vi "rszvl_core_global.vi"() -> ()   [LabVIEW 2014]
panel:
  in  "Supported Models":string[](array[string])=["ZVL", "ZNL"]
  in  "Repeated Capabilities":T1(array[cluster])=[{"repCapName"="Marker", "identifiers"=["M1", "M2", "M3", "M4"], "cmdValues"=["1", "2", "3", "4"]}, {"repCapName"="Default", "identifiers"=["DEF1", "DEF2", "DEF3"], "cmdValues"=["1", "2", "3"]}, {"repCapName"="Destination", "identifiers"=["DE1", "DE2"], "cmdValues"=["1", "2"]}, {"repCapName"="CMAP", "identifiers"=["CM1", "CM2", "CM3", "CM4", "CM5", "CM6", "CM7", "CM8", "CM9", "CM10", "CM11", "CM12", "CM13", "CM14", "CM15", "CM16", "CM17", "CM18", "CM19", "CM20", "CM21", "CM22", "CM23", "CM24", "CM25", "CM26", "CM27"], "cmdValues"=["1", "2", "3", "4", "5", "6", "7", "8", "9", "10", "11", "12", "13", "14", "15", "16", "17", "18", "19", "20", "21", "22", "23", "24", "25", "26", "27"]}, {"repCapName"="Limit", "identifiers"=["L1", "L2", "L3", "L4", "L5", "L6", "L7", "L8"], "cmdValues"=["1", "2", "3", "4", "5", "6", "7", "8"]}, {"repCapName"="DeltaMarker", "identifiers"=["DM1", "DM2", "DM3", "DM4"], "cmdValues"=["1", "2", "3", "4"]}, {"repCapName"="Trace", "identifiers"=["TR1", "TR2", "TR3", "TR4", "TR5", "TR6", "TR7", "TR8", "TR9", "TR10", "TR11", "TR12", "TR13", "TR14", "TR15", "TR16", "TR17", "TR18", "TR19", "TR20"], "cmdValues"=["1", "2", "3", "4", "5", "6", "7", "8", "9", "10", "11", "12", "13", "14", "15", "16", "17", "18", "19", "20"]}, {"repCapName"="Line", "identifiers"=["L1", "L2"], "cmdValues"=["1", "2"]}, {"repCapName"="Channel", "identifiers"=["CH1", "CH2", "CH3", "CH4", "CH5", "CH6", "CH7", "CH8", "CH9", "CH10", "CH11", "CH12", "CH13", "CH14", "CH15", "CH16", "CH17", "CH18", "CH19", "CH20"], "cmdValues"=["1", "2", "3", "4", "5", "6", "7", "8", "9", "10", "11", "12", "13", "14", "15", "16", "17", "18", "19", "20"]}, {"repCapName"="StatisticMeasType", "identifiers"=["StatMean", "StatPeak", "StatCrestFactor"], "cmdValues"=["MEAN", "PEAK", "CFAC"]}, {"repCapName"="DiagramArea", "identifiers"=["DA1", "DA2", "DA3", "DA4", "DA5", "DA6", "DA7", "DA8", "DA9", "DA10"], "cmdValues"=["1", "2", "3", "4", "5", "6", "7", "8", "9", "10"]}, {"repCapName"="Segment", "identifiers"=["SEG1", "SEG2", "SEG3", "SEG4", "SEG5", "SEG6", "SEG7", "SEG8", "SEG9", "SEG10", "SEG11", "SEG12", "SEG13", "SEG14", "SEG15", "SEG16", "SEG17", "SEG18", "SEG19", "SEG20"], "cmdValues"=["1", "2", "3", "4", "5", "6", "7", "8", "9", "10", "11", "12", "13", "14", "15", "16", "17", "18", "19", "20"]}, {"repCapName"="Port", "identifiers"=["P1", "P2", "P3", "P4", "P5", "P6", "P7", "P8", "P9", "P10"], "cmdValues"=["1", "2", "3", "4", "5", "6", "7", "8", "9", "10"]}, {"repCapName"="NWAMarker", "identifiers"=["MAR1", "MAR2", "MAR3", "MAR4", "MAR5", "MAR6", "MAR7", "MAR8", "MAR9", "MAR10"], "cmdValues"=["1", "2", "3", "4", "5", "6", "7", "8", "9", "10"]}, {"repCapName"="FMOffsetResult", "identifiers"=["FMOffImm", "FMOffAver"], "cmdValues"=["IMM", "AVER"]}, {"repCapName"="ResultDetector", "identifiers"=["ResDetPosPeak", "ResDetNegPeak", "ResDetAverPeak", "ResDetRMS"], "cmdValues"=["PPE", "MPE", "MIDD", "RMS"]}, {"repCapName"="ModifStopStart", "identifiers"=["Stop", "Start"], "cmdValues"=["STOP", "START"]}, {"repCapName"="WiMSegment", "identifiers"=["WSEG1", "WSEG2", "WSEG3"], "cmdValues"=["1", "2", "3"]}, {"repCapName"="Bitmap", "identifiers"=["B1", "B2", "B3", "B4", "B5", "B6", "B7", "B8", "B9", "B10", "B11", "B12", "B13", "B14", "B15", "B16", "B17", "B18"], "cmdValues"=["1", "2", "3", "4", "5", "6", "7", "8", "9", "10", "11", "12", "13", "14", "15", "16", "17", "18"]}, {"repCapName"="Zone", "identifiers"=["Z1", "Z2", "Z3", "Z4", "Z5", "Z6", "Z7", "Z8", "Z9", "Z10", "Z11", "Z12", "Z13", "Z14", "Z15", "Z16", "Z17", "Z18", "Z19", "Z20", "Z21", "Z22", "Z23", "Z24", "Z25", "Z26"], "cmdValues"=["1", "2", "3", "4", "5", "6", "7", "8", "9", "10", "11", "12", "13", "14", "15", "16", "17", "18", "19", "20", "21", "22", "23", "24", "25", "26"]}, {"repCapName"="Burst", "identifiers"=["BU1", "BU2", "BU3", "BU4", "BU5", "BU6", "BU7", "BU8", "BU9", "BU10", "BU11", "BU12", "BU13", "BU14", "BU15", "BU16", "BU17", "BU18", "BU19", "BU20", "BU21", "BU22", "BU23", "BU24", "BU25", "BU26", "BU27", "BU28", "BU29", "BU30", "BU31", "BU32"], "cmdValues"=["1", "2", "3", "4", "5", "6", "7", "8", "9", "10", "11", "12", "13", "14", "15", "16", "17", "18", "19", "20", "21", "22", "23", "24", "25", "26", "27", "28", "29", "30", "31", "32"]}, {"repCapName"="AnalogModulation", "identifiers"=["AnalogAM", "AnalogFM", "AnalogPM"], "cmdValues"=["AM", "FM", "PM"]}, {"repCapName"="BtoRtpTimePacketSection", "identifiers"=["SECTION_TIME_GFSK", "SECTION_TIME_DPSK"], "cmdValues"=["GAV", "DAV"]}, {"repCapName"="ModifMinMaxAver", "identifiers"=["Min", "Max", "Aver"], "cmdValues"=["MIN", "MAX", "AVER"]}, {"repCapName"="Frequency", "identifiers"=["F1", "F2"], "cmdValues"=["1", "2"]}, {"repCapName"="ModifLowUpp", "identifiers"=["Low", "Upp"], "cmdValues"=["LOW", "UPP"]}, {"repCapName"="BtoRtpPacketSection", "identifiers"=["SECTION_GFSK", "SECTION_DPSK"], "cmdValues"=["GFSK", "DPSK"]}, {"repCapName"="ModifAboveBelow", "identifiers"=["Peak", "Above", "Below", "Next"], "cmdValues"=["PEAK", "ABOV", "BEL", "NEXT"]}, {"repCapName"="InputOutput", "identifiers"=["Inp", "Out"], "cmdValues"=["INP", "OUTP"]}, {"repCapName"="NoiseTraceMemory", "identifiers"=["MEM1", "MEM2", "MEM3"], "cmdValues"=["1", "2", "3"]}, {"repCapName"="Alternate", "identifiers"=["A1", "A2", "A3", "A4"], "cmdValues"=["1", "2", "3", "4"]}, {"repCapName"="3GPPChannel", "identifiers"=["Cpich", "Pccpch"], "cmdValues"=["CPIC", "PCCP"]}, {"repCapName"="WiMAXBurstMeasurement", "identifiers"=["Carrier", "Burst", "Symbol"], "cmdValues"=["CARR", "BURS", "SYMB"]}, {"repCapName"="WiMAXMeasurement", "identifiers"=["Constellation", "Bitstream"], "cmdValues"=["CONS", "STAT:BSTR"]}, {"repCapName"="Window", "identifiers"=["Win1", "Win2"], "cmdValues"=["1", "2"]}, {"repCapName"="AtvCarrier", "identifiers"=["CN", "CSO", "CTB"], "cmdValues"=["CN", "CSO", "CTB"]}, {"repCapName"="AtvSoundCarrier", "identifiers"=["SC1", "SC2"], "cmdValues"=["S1", "S2"]}, {"repCapName"="AtvVisionModulResult", "identifiers"=["VisCarrPow", "ResPicture", "Depth"], "cmdValues"=["VCP", "RPC", "MDEP"]}, {"repCapName"="AtvCarrierResult", "identifiers"=["RefPow", "NoiseFloorCorr", "FreqRel", "CR", "NoiseRefBw"], "cmdValues"=["RPOW", "NFC", "MFR", "", "NRBW"]}, {"repCapName"="DtvErrorMeas", "identifiers"=["EVMPeak", "EVMRms", "MERPeak", "MERRms"], "cmdValues"=["EVMP", "EVMR", "MERP", "MERR"]}, {"repCapName"="DtvShoulderAtt", "identifiers"=["SAttLow", "SAttUpp"], "cmdValues"=["SAL", "SAUP"]}]
  in  "Attributes":T2(array[cluster])=[{"Level"=1, "Descriptive Name"="Basic Operation", "Class Only"=TRUE, "Data Type"=0, "Access"=0, "Identifier"="", "Range Table"="", "Command"="", "Read Callback"="", "Write Callback"="", "Range Callback"="", "Check Callback"="", "Rngtable Callback"="", "Coerce Callback"="", "User Callback"="", "Supported Models"="", "Instrument Options"="", "Repeated Capabilities"="", "Restricted Repeated Capabilities"="", "Help"="(1) Amplitude Units:\nSpecifies the amplitude units for input, output and display amplitude.\n\n(2) Instrument Mode:\nThis attribute switches between the measurement modes by means of text parameters.\n\n(3) Attenuation:\nThis attribute sets the input attenuator. To protect the input mixer against damage from overloads, the setting 0 dB can be obtained by entering numerals, not by using the command DEC.\nThe attenuation can be set in 5 dB steps. If the defined reference level cannot be set for the set RF attenuation, the reference level will be adjusted accordingly.\nIn the default state with Spectrum Analyzer mode, the attenuation set on the step attenuator is coupled to the reference level of the instrument. If the attenuation is programmed directly, the coupling to the reference level is switched off.\n\n(4) Attenuation Auto:\nEnables or disables auto attenuation.\n\n(5) Frequency Start:\nSpecifies the left edge of the frequency domain in Hertz. This is used in conjunction with the RSZVL_ATTR_FREQUENCY_STOP Stop attribute to define the frequency domain. If the RSZVL_ATTR_FREQUENCY_START attribute value is equal to the RSZVL_ATTR_FREQUENCY_STOP attribute value then the spectrum analyzers horizontal attributes are in time-domain.\n\n(6) Frequency Stop:\nSpecifies the right edge of the frequency domain in Hertz. This is used in conjunction with the RSZVL_ATTR_FREQUENCY_START attribute to define the frequency domain. If the RSZVL_ATTR_FREQUENCY_START attribute value is equal to the RSZVL_ATTR_FREQUENCY_STOP attribute value then the spectrum analyzers horizontal attributes are in time-domain.\n\n(7) Frequency Offset:\nThis attribute sets the frequency offset of the instrument.\n\n(8) Center Frequency:\nThe attribute defines the center frequency of the analyzer or the measuring frequency for span = 0.\n\n(9) Center Frequency Step:\nThis attribute defines the step width of the center frequency.\n\n(10) Center Frequency Step Auto:\nThis attribute couples the step size of the center frequency to the span (ON) or sets the value of the center frequency entered via [SENSe<1|2>:]FREQuency:CENTer:STEP (OFF).\n\n(11) Center Frequency Coupling:\nThis attribute couples the step width of the center frequency to span (span >0) or to the resolution bandwidth (span = 0) or cancels the couplings.\n\n(12) Center Frequency Coupling Factor:\nThis attribute couples the step width of the center frequency with a factor to the span (span >0) or to the resolution bandwidth (span = 0).\n\n(13) Frequency Span:\nThis attribute defines the frequency span in the analyzer mode.\n\n(14) Full Frequency Span:\nThis attribute sets the frequency span in the analyzer mode to its maximum.\n\n(15) Frequency Mode:\nThis attribute switches between frequency domain (SWEep) and time domain (CW | FIXed) in the analyzer mode. For CW and FIXed, the frequency setting is via command FREQuency:CENTer. In the SWEep mode, the setting is via commands FREQuency:STARt, STOP, CENTer and SPAN.\n\n(16) Input Impedance:\nThis attribute the nominal input impedance of the instrument. The set impedance is taken into account in all level indications of results.\n\n(17) Number of Sweeps:\nThis attribute defines the number of sweeps started with single sweep, which are used for calculating the average or maximum value. In average mode, the value 0 defines a continuous averaging of measurement data over 10 sweeps.\n\n(18) Reference Level:\nThis attribute configures the reference level for the signal analyzer mode.\n\n\n(19) Reference Level Offset:\nThis attribute defines the offset of the reference level.\n\n(20) Resolution Bandwidth:\nThis attribute defines the analyzer's resolution bandwidth.\n\n(21) Resolution Bandwidth Auto:\nIn SPECTRUM mode, this attribute either automatically couples the resolution bandwidth of the instrument to the span or cancels the coupling.\nIn FM DEMOD mode, this attribute either automatically couples the IF bandwidth of the instrument to the demodulation bandwidth or cancels the coupling (BWRBW = 10 * BWDemod).\nIn FM DEMOD mode, the coupling refers to the demodulation bandwidth (BWRBW = 10 * BWDemod). The automatic coupling adapts the resolution bandwidth to the currently set frequency span according to the relationship between frequency span and resolution bandwidth. The 6 dB bandwidths 200 Hz, 9 kHz and 120 kHz and the channel filters available from Version 1.10 are not set by the automatic coupling.\n\nNote: This attribute is not available for GSM/EDGE measurements modulation accuracy (MAC), phase/frequency error (PFE) and power versus time (PVT). During these measurements the bandwidth is selected due to GSM standard.\n\n(22) Resolution Bandwidth Ratio:\nThis attribute defines the ratio resolution bandwidth (Hz) / span (Hz). The ratio to be entered is reciprocal to the ratio span/RBW used in manual control.\n\n(23) Sweep Mode:\nThis attribute determines whether the trigger system is continuously initiated (continuous) or performs single measurements (single).\nIn the spectrum analysis mode, this setting refers to the sweep sequence (switching between continuous/single sweep).\n\n(24) Sweep Time:\nThis attribute defines the sweep time.\n\n(25) Sweep Time Auto:\nThis attribute controls the automatic coupling of the sweep time to the frequency span and bandwidth settings.\n\n(26) Sweep Points:\nThis attribute defines the number of measurement points for one sweep run.\n\n(27) Get Sweep Count Current:\nThis attribute returns the current number of started sweeps. A sweep count value should be set and the device should be in single sweep mode.\n\n(28) Vertical Scale:\nThis attribute toggles between linear and logarithmic display.\n\n(29) Video Bandwidth:\nThis attribute defines the instrument's video bandwidth.\n\n(30) Video Bandwidth Auto:\nThis attribute either automatically couples the instrument's video bandwidth to the resolution bandwidth or cancels the coupling.\n\n(31) Video Bandwidth Ratio:\nThis attribute defines the ratio video bandwidth (Hz) / resolution bandwidth (Hz). The ratio to be entered is reciprocal to the ratio RBW/VBW used in manual control.\n\n(32) Low-Level Measurement (Class):\nThis class contains attributes for initiate and abort measurement.\n\n(1) Abort:\nThis attribute aborts a current measurement and resets the trigger system.\n\n(2) Initiate:\nThis attribute initiates a new sweep.\nIn single sweep mode, synchronization to the end of the indicated number of measurements is achieved with the command *OPC. In continuous-sweep mode, synchronization to the sweep end is not possible since the overall measurement never ends.\n\n(3) Initiate Continuous:\nThis attribute determines whether the trigger system is continuously initiated (continuous) or performs single measurements (single).\nIn the spectrum analysis mode, this setting refers to the sweep sequence (switching between continuous/single sweep).\n\n(4) Send Software Trigger:\nThis attribute sends a software trigger to the instrument.\n\n(5) Continue Measurement:\nThis attribute continues a stopped measurement at the current position in single sweep mode. The function is useful especially for trace functions MAXHold, MINHold and AVERage if the previous results are not to be cleared with Sweep Count > 0 or Average Count > 0 on restarting the measurement (INIT:IMMediate resets the previous results on restarting the measurement).\nThe single-sweep mode is automatically switched on. Synchronization to the end of the indicated number of measurements can then be performed with the command *OPC, *OPC? or *WAI. In the continuous-sweep mode, synchronization to the sweep end is not possible since the overall measurement never ends.\n\n\n\n(33) Average (Class):\nThis subsystem calculates the average of the acquired data.\n\n(1) Averaging State:\nThis attribute switches on or off the average calculation for the selected trace.\n\n(2) Averaging Type:\nThis attribute selects the type of average function. If Video is selected, the logarithmic power is averaged and, if Linear is selected, the power values are averaged before they are converted to logarithmic values. The type of average calculation is equally set for all traces\n\n(3) Averaging Count:\nThis attribute defines the number of measurements which contribute to the average value.\nIt should be noted that continuous averaging will be performed after the indicated number has been reached in continuous sweep mode.\nIn single sweep mode, the sweep is stopped as soon as the indicated number of measurements (sweeps) is reached. Synchronization to the end of the indicated number of measurements is only possible in single sweep mode.\n\n(4) Averaging Count Auto:\nThis attribute is implemented only for reasons of compatibility with the FSP family. It selects a suitable number of counts for the selected measurement type.\n\n\n\n(34) Bandwidth (Class):\nThis class contains attributes configuring resolution and video bandwidth.\n\n(1) Resolution Bandwidth Filter Type:\nThis attribute sets the filter type for the resolution bandwidth.\n\n(2) Video Bandwidth Filter Type:\nThis attribute selects the position of the video filter in the signal path, provided that the resolution bandwidth is <=100 kHz:\n\n(35) Trace (Class):\nTrace settings and configuration.\n\n(1) Trace State:\nThis attribute switches on or off the display of the corresponding trace.\n\n(2) Trace Reset Behavior:\nThis attribute specifies whether or not the traces with peak or minimum value detection are reset after specific parameter changes.\n\n(3) Trace Type:\nThis attribute defines the type of display and the evaluation of the traces. WRITE corresponds to the Clr/Write mode of manual operation. The trace is switched off (= BLANK in manual operation) with DISP:WIND:TRAC:STAT OFF.\n\n(4) Trace Math State:\nThis attribute switches the mathematical relation of traces on or off.\n\n(5) Trace Math Position:\nThis attribute defines the position of the result of the trace mathematics. The indication is in % of the screen height, with 100% corresponding to the upper diagram border.\n\n(6) Detector Type:\nSpecifies the detection method used to capture and process the signal. This governs the data acquisition for a particular sweep, but does not have any control over how multiple sweeps are processed.\n\n(7) Detector Type Auto:\nEnables the auto detector.\n\n(36) Calibration (Class):\n(1) Calibration:\nThis attribute initiates the acquisition of system error correction data. A 0 is returned if the acquisition was successful.\n\n(2) Calibration Abort:\nThis atribute aborts the acquisition of correction data and restores the last complete correction data set.\n\n(3) Calibration Result Query:\nThis attribute outputs the results of the correction data acquisition.\n\n(4) Calibration State:\nThis attribute determines whether the current calibration data are taken into account by the instrument (ON) or not (OFF).\n\n\n\n(37) User Port (Class):\n(1) User Ports State:\nThis attribute toggles the control lines of the user ports between INPut and OUTPut. With ON, the user port is switched to INPut, with OFF to OUTPut.\n\n(2) User Ports Control Lines:\nThis attribute queries the control lines of the user ports.\n\n(3) User Ports Output Control Lines:\nThis attribute sets the control lines of the user ports. The user port is written to with the given binary pattern. If the user port is programmed to INPut instead of OUTPut, the output value is temporarily stored.", "Flags"={"OPC Wait"=FALSE, "Dont check status"=FALSE, "*WAI"=FALSE}, "Check Status Callback"=""}, {"Level"=2, "Descriptive Name"="Amplitude Units", "Class Only"=FALSE, "Data Type"=0, "Access"=2, "Identifier"="RSZVL_ATTR_AMPLITUDE_UNITS", "Range Table"="rszvl_rngAmplitudeUnitsRangeTable", "Command"="UNIT:POW", "Read Callback"="", "Write Callback"="", "Range Callback"="", "Check Callback"="", "Rngtable Callback"="", "Coerce Callback"="", "User Callback"="", "Supported Models"="", "Instrument Options"="", "Repeated Capabilities"="", "Restricted Repeated Capabilities"="", "Help"="Specifies the amplitude units for input, output and display amplitude.\n\nAvailable Repeated Capabilities:\nNone\n\nRemote-control command(s):\nUNIT<1|2>:POWer DBM | DBPW | WATT | DBUV | DBMV | VOLT | DBUA | AMPere", "Flags"={"OPC Wait"=FALSE, "Dont check status"=FALSE, "*WAI"=FALSE}, "Check Status Callback"=""}, {"Level"=2, "Descriptive Name"="Instrument Mode", "Class Only"=FALSE, "Data Type"=0, "Access"=2, "Identifier"="RSZVL_ATTR_INSTR_MODE", "Range Table"="rszvl_rngInstrMode", "Command"="INST:SEL", "Read Callback"="", "Write Callback"="", "Range Callback"="", "Check Callback"="", "Rngtable Callback"="", "Coerce Callback"="", "User Callback"="", "Supported Models"="", "Instrument Options"="", "Repeated Capabilities"="", "Restricted Repeated Capabilities"="", "Help"="This attribute switches between the measurement modes by means of text parameters.\n\nAvailable Repeated Capabilities:\nNone\n\nRemote-control command(s):\nINSTrument[:SELect] NWA | SAN | NOISe | BWCD | WLAN | WiMAX | ADEM | BTO | CATV", "Flags"={"OPC Wait"=FALSE, "Dont check status"=FALSE, "*WAI"=FALSE}, "Check Status Callback"=""}, {"Level"=2, "Descriptive Name"="Attenuation", "Class Only"=FALSE, "Data Type"=1, "Access"=2, "Identifier"="RSZVL_ATTR_ATTENUATION", "Range Table"="rszvl_rngAttenuationRangeTable", "Command"="INP:ATT", "Read Callback"="", "Write Callback"="", "Range Callback"="", "Check Callback"="", "Rngtable Callback"="", "Coerce Callback"="", "User Callback"="", "Supported Models"="", "Instrument Options"="", "Repeated Capabilities"="", "Restricted Repeated Capabilities"="", "Help"="This attribute sets the input attenuator. To protect the input mixer against damage from overloads, the setting 0 dB can be obtained by entering numerals, not by using the command DEC.\nThe attenuation can be set in 5 dB steps. If the defined reference level cannot be set for the set RF attenuation, the reference level will be adjusted accordingly.\nIn the default state with Spectrum Analyzer mode, the attenuation set on the step attenuator is coupled to the reference level of the instrument. If the attenuation is programmed directly, the coupling to the reference level is switched off.\n\nAvailable Repeated Capabilities:\nNone\n\nRemote-control command(s):\nINPut<1|2>:ATTenuation", "Flags"={"OPC Wait"=FALSE, "Dont check status"=FALSE, "*WAI"=FALSE}, "Check Status Callback"=""}, {"Level"=2, "Descriptive Name"="Attenuation Auto", "Class Only"=FALSE, "Data Type"=3, "Access"=2, "Identifier"="RSZVL_ATTR_ATTENUATION_AUTO", "Range Table"="", "Command"="INP:ATT:AUTO", "Read Callback"="", "Write Callback"="", "Range Callback"="", "Check Callback"="", "Rngtable Callback"="", "Coerce Callback"="", "User Callback"="", "Supported Models"="", "Instrument Options"="", "Repeated Capabilities"="", "Restricted Repeated Capabilities"="", "Help"="Enables or disables auto attenuation.\n\nAvailable Repeated Capabilities:\nNone\n\nRemote-control command(s):\nINPut<1|2>:ATTenuation:AUTO ON | OFF", "Flags"={"OPC Wait"=FALSE, "Dont check status"=FALSE, "*WAI"=FALSE}, "Check Status Callback"=""}, {"Level"=2, "Descriptive Name"="Frequency Start", "Class Only"=FALSE, "Data Type"=1, "Access"=2, "Identifier"="RSZVL_ATTR_FREQUENCY_START", "Range Table"="", "Command"="SENS:FREQ:STAR", "Read Callback"="", "Write Callback"="", "Range Callback"="", "Check Callback"="", "Rngtable Callback"="", "Coerce Callback"="", "User Callback"="", "Supported Models"="", "Instrument Options"="", "Repeated Capabilities"="", "Restricted Repeated Capabilities"="", "Help"="Specifies the left edge of the frequency domain in Hertz. This is used in conjunction with the RSZVL_ATTR_FREQUENCY_STOP Stop attribute to define the frequency domain. If the RSZVL_ATTR_FREQUENCY_START attribute value is equal to the RSZVL_ATTR_FREQUENCY_STOP attribute value then the spectrum analyzers horizontal attributes are in time-domain.\n\nAvailable Repeated Capabilities:\nNone\n\nRemote-control command(s):\n[SENSe<1|2>]:FREQuency:STARt", "Flags"={"OPC Wait"=FALSE, "Dont check status"=FALSE, "*WAI"=FALSE}, "Check Status Callback"=""}, {"Level"=2, "Descriptive Name"="Frequency Stop", "Class Only"=FALSE, "Data Type"=1, "Access"=2, "Identifier"="RSZVL_ATTR_FREQUENCY_STOP", "Range Table"="", "Command"="SENS:FREQ:STOP", "Read Callback"="", "Write Callback"="", "Range Callback"="", "Check Callback"="", "Rngtable Callback"="", "Coerce Callback"="", "User Callback"="", "Supported Models"="", "Instrument Options"="", "Repeated Capabilities"="", "Restricted Repeated Capabilities"="", "Help"="Specifies the right edge of the frequency domain in Hertz. This is used in conjunction with the RSZVL_ATTR_FREQUENCY_START attribute to define the frequency domain. If the RSZVL_ATTR_FREQUENCY_START attribute value is equal to the RSZVL_ATTR_FREQUENCY_STOP attribute value then the spectrum analyzers horizontal attributes are in time-domain.\n\nAvailable Repeated Capabilities:\nNone\n\nRemote-control command(s):\n[SENSe<1|2>]:FREQuency:STOP", "Flags"={"OPC Wait"=FALSE, "Dont check status"=FALSE, "*WAI"=FALSE}, "Check Status Callback"=""}, {"Level"=2, "Descriptive Name"="Frequency Offset", "Class Only"=FALSE, "Data Type"=1, "Access"=2, "Identifier"="RSZVL_ATTR_FREQUENCY_OFFSET", "Range Table"="rszvl_rngFreqOffset", "Command"="SENS:FREQ:OFFS", "Read Callback"="", "Write Callback"="", "Range Callback"="", "Check Callback"="", "Rngtable Callback"="", "Coerce Callback"="", "User Callback"="", "Supported Models"="", "Instrument Options"="", "Repeated Capabilities"="", "Restricted Repeated Capabilities"="", "Help"="This attribute sets the frequency offset of the instrument.\n\nAvailable Repeated Capabilities:\nNone\n\nRemote-control command(s):\n[SENSe<1|2>:]FREQuency:OFFSet", "Flags"={"OPC Wait"=FALSE, "Dont check status"=FALSE, "*WAI"=FALSE}, "Check Status Callback"=""}, {"Level"=2, "Descriptive Name"="Center Frequency", "Class Only"=FALSE, "Data Type"=1, "Access"=2, "Identifier"="RSZVL_ATTR_FREQUENCY_CENTER", "Range Table"="", "Command"="SENS:FREQ:CENT", "Read Callback"="", "Write Callback"="", "Range Callback"="", "Check Callback"="", "Rngtable Callback"="", "Coerce Callback"="", "User Callback"="", "Supported Models"="", "Instrument Options"="", "Repeated Capabilities"="", "Restricted Repeated Capabilities"="", "Help"="The attribute defines the center frequency of the analyzer or the measuring frequency for span = 0.\n\nAvailable Repeated Capabilities:\nNone\n\nRemote-control command(s):\n[SENSe<1|2>:]FREQuency:CENTer", "Flags"={"OPC Wait"=FALSE, "Dont check status"=FALSE, "*WAI"=FALSE}, "Check Status Callback"=""}, {"Level"=2, "Descriptive Name"="Center Frequency Step", "Class Only"=FALSE, "Data Type"=1, "Access"=2, "Identifier"="RSZVL_ATTR_FREQUENCY_CENTER_STEP", "Range Table"="", "Command"="SENS:FREQ:CENT:STEP", "Read Callback"="", "Write Callback"="", "Range Callback"="", "Check Callback"="", "Rngtable Callback"="", "Coerce Callback"="", "User Callback"="", "Supported Models"="", "Instrument Options"="", "Repeated Capabilities"="", "Restricted Repeated Capabilities"="", "Help"="This attribute defines the step width of the center frequency.\n\nAvailable Repeated Capabilities:\nNone\n\nRemote-control command(s):\n[SENSe<1|2>:]FREQuency:CENTer:STEP", "Flags"={"OPC Wait"=FALSE, "Dont check status"=FALSE, "*WAI"=FALSE}, "Check Status Callback"=""}, {"Level"=2, "Descriptive Name"="Center Frequency Step Auto", "Class Only"=FALSE, "Data Type"=3, "Access"=2, "Identifier"="RSZVL_ATTR_FREQUENCY_STEP_AUTO", "Range Table"="", "Command"="SENS:FREQ:CENT:STEP:AUTO", "Read Callback"="", "Write Callback"="", "Range Callback"="", "Check Callback"="", "Rngtable Callback"="", "Coerce Callback"="", "User Callback"="", "Supported Models"="", "Instrument Options"="", "Repeated Capabilities"="", "Restricted Repeated Capabilities"="", "Help"="This attribute couples the step size of the center frequency to the span (ON) or sets the value of the center frequency entered via [SENSe<1|2>:]FREQuency:CENTer:STEP (OFF).\n\nAvailable Repeated Capabilities:\nNone\n\nRemote-control command(s):\n[SENSe<1|2>:]FREQuency:CENTer:STEP:AUTO ON | OFF", "Flags"={"OPC Wait"=FALSE, "Dont check status"=FALSE, "*WAI"=FALSE}, "Check Status Callback"=""}, {"Level"=2, "Descriptive Name"="Center Frequency Coupling", "Class Only"=FALSE, "Data Type"=0, "Access"=2, "Identifier"="RSZVL_ATTR_FREQUENCY_CENTER_LINK", "Range Table"="rszvl_rngFreqCentLink", "Command"="SENS:FREQ:CENT:STEP:LINK", "Read Callback"="", "Write Callback"="", "Range Callback"="", "Check Callback"="", "Rngtable Callback"="", "Coerce Callback"="", "User Callback"="", "Supported Models"="", "Instrument Options"="", "Repeated Capabilities"="", "Restricted Repeated Capabilities"="", "Help"="This attribute couples the step width of the center frequency to span (span >0) or to the resolution bandwidth (span = 0) or cancels the couplings.\n\nAvailable Repeated Capabilities:\nNone\n\nRemote-control command(s):\n[SENSe<1|2>:]FREQuency:CENTer:STEP:LINK SPAN | RBW | OFF", "Flags"={"OPC Wait"=FALSE, "Dont check status"=FALSE, "*WAI"=FALSE}, "Check Status Callback"=""}, {"Level"=2, "Descriptive Name"="Center Frequency Coupling Factor", "Class Only"=FALSE, "Data Type"=0, "Access"=2, "Identifier"="RSZVL_ATTR_FREQUENCY_CENTER_LINK_FACTOR", "Range Table"="rszvl_rngLinkFactor", "Command"="SENS:FREQ:CENT:STEP:LINK:FACT", "Read Callback"="", "Write Callback"="", "Range Callback"="", "Check Callback"="", "Rngtable Callback"="", "Coerce Callback"="", "User Callback"="", "Supported Models"="", "Instrument Options"="", "Repeated Capabilities"="", "Restricted Repeated Capabilities"="", "Help"="This attribute couples the step width of the center frequency with a factor to the span (span >0) or to the resolution bandwidth (span = 0).\n\nAvailable Repeated Capabilities:\nNone\n\nRemote-control command(s):\n[SENSe<1|2>:]FREQuency:CENTer:STEP:LINK:FACTor", "Flags"={"OPC Wait"=FALSE, "Dont check status"=FALSE, "*WAI"=FALSE}, "Check Status Callback"=""}, {"Level"=2, "Descriptive Name"="Frequency Span", "Class Only"=FALSE, "Data Type"=1, "Access"=2, "Identifier"="RSZVL_ATTR_FREQUENCY_SPAN", "Range Table"="", "Command"="SENS:FREQ:SPAN", "Read Callback"="", "Write Callback"="", "Range Callback"="", "Check Callback"="", "Rngtable Callback"="", "Coerce Callback"="", "User Callback"="", "Supported Models"="", "Instrument Options"="", "Repeated Capabilities"="", "Restricted Repeated Capabilities"="", "Help"="This attribute defines the frequency span in the analyzer mode.\n\nAvailable Repeated Capabilities:\nNone\n\nRemote-control command(s):\n[SENSe<1|2>:]FREQuency:SPAN", "Flags"={"OPC Wait"=FALSE, "Dont check status"=FALSE, "*WAI"=FALSE}, "Check Status Callback"=""}, {"Level"=2, "Descriptive Name"="Full Frequency Span", "Class Only"=FALSE, "Data Type"=4, "Access"=1, "Identifier"="RSZVL_ATTR_FREQUENCY_SPAN_FULL", "Range Table"="", "Command"="SENS:FREQ:SPAN:FULL", "Read Callback"="", "Write Callback"="", "Range Callback"="", "Check Callback"="", "Rngtable Callback"="", "Coerce Callback"="", "User Callback"="", "Supported Models"="", "Instrument Options"="", "Repeated Capabilities"="", "Restricted Repeated Capabilities"="", "Help"="This attribute sets the frequency span in the analyzer mode to its maximum.\n\nAvailable Repeated Capabilities:\nNone\n\nRemote-control command(s):\n[SENSe<1|2>:]FREQuency:SPAN:FULL", "Flags"={"OPC Wait"=FALSE, "Dont check status"=FALSE, "*WAI"=FALSE}, "Check Status Callback"=""}, {"Level"=2, "Descriptive Name"="Frequency Mode", "Class Only"=FALSE, "Data Type"=0, "Access"=2, "Identifier"="RSZVL_ATTR_FREQUENCY_MODE", "Range Table"="rszvl_rngFreqMode", "Command"="SENS:FREQ:MODE", "Read Callback"="", "Write Callback"="", "Range Callback"="", "Check Callback"="", "Rngtable Callback"="", "Coerce Callback"="", "User Callback"="", "Supported Models"="", "Instrument Options"="", "Repeated Capabilities"="", "Restricted Repeated Capabilities"="", "Help"="This attribute switches between frequency domain (SWEep) and time domain (CW | FIXed) in the analyzer mode. For CW and FIXed, the frequency setting is via command FREQuency:CENTer. In the SWEep mode, the setting is via commands FREQuency:STARt, STOP, CENTer and SPAN.\n\nAvailable Repeated Capabilities:\nNone\n\nRemote-control command(s):\n[SENSe<1|2>:]FREQuency:MODE CW | FIXed | SWEep", "Flags"={"OPC Wait"=FALSE, "Dont check status"=FALSE, "*WAI"=FALSE}, "Check Status Callback"=""}, {"Level"=2, "Descriptive Name"="Input Impedance", "Class Only"=FALSE, "Data Type"=1, "Access"=2, "Identifier"="RSZVL_ATTR_INPUT_IMPEDANCE", "Range Table"="rszvl_rngInputImpedance", "Command"="INP:IMP", "Read Callback"="", "Write Callback"="", "Range Callback"="", "Check Callback"="", "Rngtable Callback"="", "Coerce Callback"="", "User Callback"="", "Supported Models"="", "Instrument Options"="", "Repeated Capabilities"="", "Restricted Repeated Capabilities"="", "Help"="This attribute the nominal input impedance of the instrument. The set impedance is taken into account in all level indications of results.\n\nAvailable Repeated Capabilities:\nNone\n\nRemote-control command(s):\nINPut<1|2>:IMPedance", "Flags"={"OPC Wait"=FALSE, "Dont check status"=FALSE, "*WAI"=FALSE}, "Check Status Callback"=""}, {"Level"=2, "Descriptive Name"="Number of Sweeps", "Class Only"=FALSE, "Data Type"=0, "Access"=2, "Identifier"="RSZVL_ATTR_NUMBER_OF_SWEEPS", "Range Table"="rszvl_rngSweepCount", "Command"="SENS:SWE:COUN", "Read Callback"="", "Write Callback"="", "Range Callback"="", "Check Callback"="", "Rngtable Callback"="", "Coerce Callback"="", "User Callback"="", "Supported Models"="", "Instrument Options"="", "Repeated Capabilities"="", "Restricted Repeated Capabilities"="", "Help"="This attribute defines the number of sweeps started with single sweep, which are used for calculating the average or maximum value. In average mode, the value 0 defines a continuous averaging of measurement data over 10 sweeps.\n\nAvailable Repeated Capabilities:\nNone\n\nRemote-control command(s):\n[SENSe<1|2>:]SWEep:COUNt", "Flags"={"OPC Wait"=FALSE, "Dont check status"=FALSE, "*WAI"=FALSE}, "Check Status Callback"=""}, {"Level"=2, "Descriptive Name"="Reference Level", "Class Only"=FALSE, "Data Type"=1, "Access"=2, "Identifier"="RSZVL_ATTR_REFERENCE_LEVEL", "Range Table"="", "Command"="DISP:WIND:TRAC:Y:RLEV", "Read Callback"="", "Write Callback"="", "Range Callback"="", "Check Callback"="", "Rngtable Callback"="", "Coerce Callback"="", "User Callback"="", "Supported Models"="", "Instrument Options"="", "Repeated Capabilities"="", "Restricted Repeated Capabilities"="", "Help"="This attribute configures the reference level for the signal analyzer mode.\n\nAvailable Repeated Capabilities:\nNone\n\nRemote-control command(s):\nDISPlay[:WINDow<1|2>]:TRACe<1 to 6>:Y[:SCALe]:RLEVel", "Flags"={"OPC Wait"=FALSE, "Dont check status"=FALSE, "*WAI"=FALSE}, "Check Status Callback"=""}, {"Level"=2, "Descriptive Name"="Reference Level Offset", "Class Only"=FALSE, "Data Type"=1, "Access"=2, "Identifier"="RSZVL_ATTR_REFERENCE_LEVEL_OFFSET", "Range Table"="rszvl_rngRefLevel", "Command"="DISP:WIND:TRAC:Y:RLEV:OFFS", "Read Callback"="", "Write Callback"="", "Range Callback"="", "Check Callback"="", "Rngtable Callback"="", "Coerce Callback"="", "User Callback"="", "Supported Models"="", "Instrument Options"="", "Repeated Capabilities"="", "Restricted Repeated Capabilities"="", "Help"="This attribute defines the offset of the reference level.\n\nAvailable Repeated Capabilities:\nNone\n\nRemote-control command(s):\nDISPlay[:WINDow<1|2>]:TRACe<1 to 6>:Y[:SCALe]:RLEVel:OFFSet", "Flags"={"OPC Wait"=FALSE, "Dont check status"=FALSE, "*WAI"=FALSE}, "Check Status Callback"=""}, {"Level"=2, "Descriptive Name"="Resolution Bandwidth", "Class Only"=FALSE, "Data Type"=1, "Access"=2, "Identifier"="RSZVL_ATTR_RESOLUTION_BANDWIDTH", "Range Table"="rszvl_rngRBW", "Command"="SENS:BAND", "Read Callback"="", "Write Callback"="", "Range Callback"="", "Check Callback"="", "Rngtable Callback"="", "Coerce Callback"="", "User Callback"="", "Supported Models"="", "Instrument Options"="", "Repeated Capabilities"="", "Restricted Repeated Capabilities"="", "Help"="This attribute defines the analyzer's resolution bandwidth.\n\nAvailable Repeated Capabilities:\nNone\n\nRemote-control command(s):\n[SENSe<1|2>:]BANDwidth|BWIDth[:RESolution]", "Flags"={"OPC Wait"=FALSE, "Dont check status"=FALSE, "*WAI"=FALSE}, "Check Status Callback"=""}, {"Level"=2, "Descriptive Name"="Resolution Bandwidth Auto", "Class Only"=FALSE, "Data Type"=3, "Access"=2, "Identifier"="RSZVL_ATTR_RESOLUTION_BANDWIDTH_AUTO", "Range Table"="", "Command"="SENS:BAND:AUTO", "Read Callback"="", "Write Callback"="", "Range Callback"="", "Check Callback"="", "Rngtable Callback"="", "Coerce Callback"="", "User Callback"="", "Supported Models"="", "Instrument Options"="", "Repeated Capabilities"="", "Restricted Repeated Capabilities"="", "Help"="In SPECTRUM mode, this attribute either automatically couples the resolution bandwidth of the instrument to the span or cancels the coupling.\nIn FM DEMOD mode, this attribute either automatically couples the IF bandwidth of the instrument to the demodulation bandwidth or cancels the coupling (BWRBW = 10 * BWDemod).\nIn FM DEMOD mode, the coupling refers to the demodulation bandwidth (BWRBW = 10 * BWDemod). The automatic coupling adapts the resolution bandwidth to the currently set frequency span according to the relationship between frequency span and resolution bandwidth. The 6 dB bandwidths 200 Hz, 9 kHz and 120 kHz and the channel filters available from Version 1.10 are not set by the automatic coupling.\n\nNote: This attribute is not available for GSM/EDGE measurements modulation accuracy (MAC), phase/frequency error (PFE) and power versus time (PVT). During these measurements the bandwidth is selected due to GSM standard.\n\nAvailable Repeated Capabilities:\nNone\n\nRemote-control command(s):\n[SENSe<1|2>:]BANDwidth|BWIDth[:RESolution]:AUTO", "Flags"={"OPC Wait"=FALSE, "Dont check status"=FALSE, "*WAI"=FALSE}, "Check Status Callback"=""}, {"Level"=2, "Descriptive Name"="Resolution Bandwidth Ratio", "Class Only"=FALSE, "Data Type"=1, "Access"=2, "Identifier"="RSZVL_ATTR_RESOLUTION_BANDWIDTH_RATIO", "Range Table"="rszvl_rngBandRatio", "Command"="SENS:BAND:RAT", "Read Callback"="", "Write Callback"="", "Range Callback"="", "Check Callback"="", "Rngtable Callback"="", "Coerce Callback"="", "User Callback"="", "Supported Models"="", "Instrument Options"="", "Repeated Capabilities"="", "Restricted Repeated Capabilities"="", "Help"="This attribute defines the ratio resolution bandwidth (Hz) / span (Hz). The ratio to be entered is reciprocal to the ratio span/RBW used in manual control.\n\nAvailable Repeated Capabilities:\nNone\n\nRemote-control command(s):\n[SENSe<1|2>:]BANDwidth|BWIDth[:RESolution]:RATio", "Flags"={"OPC Wait"=FALSE, "Dont check status"=FALSE, "*WAI"=FALSE}, "Check Status Callback"=""}, {"Level"=2, "Descriptive Name"="Sweep Mode", "Class Only"=FALSE, "Data Type"=3, "Access"=2, "Identifier"="RSZVL_ATTR_SWEEP_MODE_CONTINUOUS", "Range Table"="", "Command"="INIT:CONT", "Read Callback"="", "Write Callback"="", "Range Callback"="", "Check Callback"="", "Rngtable Callback"="", "Coerce Callback"="", "User Callback"="", "Supported Models"="", "Instrument Options"="", "Repeated Capabilities"="", "Restricted Repeated Capabilities"="", "Help"="This attribute determines whether the trigger system is continuously initiated (continuous) or performs single measurements (single).\nIn the spectrum analysis mode, this setting refers to the sweep sequence (switching between continuous/single sweep).\n\nAvailable Repeated Capabilities:\nNone\n\nRemote-control command(s):\nINITiate<1|2>:CONTinuous ON | OFF", "Flags"={"OPC Wait"=FALSE, "Dont check status"=FALSE, "*WAI"=FALSE}, "Check Status Callback"=""}, {"Level"=2, "Descriptive Name"="Sweep Time", "Class Only"=FALSE, "Data Type"=1, "Access"=2, "Identifier"="RSZVL_ATTR_SWEEP_TIME", "Range Table"="rszvl_rngSweepTime", "Command"="SENS:SWE:TIME", "Read Callback"="", "Write Callback"="", "Range Callback"="", "Check Callback"="", "Rngtable Callback"="", "Coerce Callback"="", "User Callback"="", "Supported Models"="", "Instrument Options"="", "Repeated Capabilities"="", "Restricted Repeated Capabilities"="", "Help"="This attribute defines the sweep time.\n\nAvailable Repeated Capabilities:\nNone\n\nRemote-control command(s):\n[SENSe<1|2>:]SWEep:TIME", "Flags"={"OPC Wait"=FALSE, "Dont check status"=FALSE, "*WAI"=FALSE}, "Check Status Callback"=""}, {"Level"=2, "Descriptive Name"="Sweep Time Auto", "Class Only"=FALSE, "Data Type"=3, "Access"=2, "Identifier"="RSZVL_ATTR_SWEEP_TIME_AUTO", "Range Table"="", "Command"="SENS:SWE:TIME:AUTO", "Read Callback"="", "Write Callback"="", "Range Callback"="", "Check Callback"="", "Rngtable Callback"="", "Coerce Callback"="", "User Callback"="", "Supported Models"="", "Instrument Options"="", "Repeated Capabilities"="", "Restricted Repeated Capabilities"="", "Help"="This attribute controls the automatic coupling of the sweep time to the frequency span and bandwidth settings.\n\nAvailable Repeated Capabilities:\nNone\n\nRemote-control command(s):\n[SENSe<1|2>:]SWEep:TIME:AUTO ON | OFF", "Flags"={"OPC Wait"=FALSE, "Dont check status"=FALSE, "*WAI"=FALSE}, "Check Status Callback"=""}, {"Level"=2, "Descriptive Name"="Sweep Points", "Class Only"=FALSE, "Data Type"=0, "Access"=2, "Identifier"="RSZVL_ATTR_SWEEP_POINTS", "Range Table"="rszvl_rngSwePoints", "Command"="SENS:SWE:POIN", "Read Callback"="", "Write Callback"="", "Range Callback"="", "Check Callback"="", "Rngtable Callback"="", "Coerce Callback"="", "User Callback"="", "Supported Models"="", "Instrument Options"="", "Repeated Capabilities"="", "Restricted Repeated Capabilities"="", "Help"="This attribute defines the number of measurement points for one sweep run.\n\nAvailable Repeated Capabilities:\nNone\n\nRemote-control command(s):\n[SENSe<1|2>:]SWEep:POINts", "Flags"={"OPC Wait"=FALSE, "Dont check status"=FALSE, "*WAI"=FALSE}, "Check Status Callback"=""}, {"Level"=2, "Descriptive Name"="Get Sweep Count Current", "Class Only"=FALSE, "Data Type"=0, "Access"=0, "Identifier"="RSZVL_ATTR_SWEEP_COUNT_CURRENT", "Range Table"="", "Command"="SENS:SWE:COUN:CURR?", "Read Callback"="", "Write Callback"="", "Range Callback"="", "Check Callback"="", "Rngtable Callback"="", "Coerce Callback"="", "User Callback"="", "Supported Models"="", "Instrument Options"="", "Repeated Capabilities"="", "Restricted Repeated Capabilities"="", "Help"="This attribute returns the current number of started sweeps. A sweep count value should be set and the device should be in single sweep mode.\n\nAvailable Repeated Capabilities:\nNone\n\nRemote-control command(s):\n[SENSe<1|2>:]SWEep:COUNt:CURRent?", "Flags"={"OPC Wait"=FALSE, "Dont check status"=FALSE, "*WAI"=FALSE}, "Check Status Callback"=""}, {"Level"=2, "Descriptive Name"="Vertical Scale", "Class Only"=FALSE, "Data Type"=0, "Access"=2, "Identifier"="RSZVL_ATTR_VERTICAL_SCALE", "Range Table"="rszvl_rngTraceSpacing", "Command"="DISP:WIND:TRAC:Y:SPAC", "Read Callback"="", "Write Callback"="", "Range Callback"="", "Check Callback"="", "Rngtable Callback"="", "Coerce Callback"="", "User Callback"="", "Supported Models"="", "Instrument Options"="", "Repeated Capabilities"="", "Restricted Repeated Capabilities"="", "Help"="This attribute toggles between linear and logarithmic display.\n\nAvailable Repeated Capabilities:\nNone\n\nRemote-control command(s):\nDISPlay[:WINDow<1|2>]:TRACe<1 to 6>:Y:SPACing LINear | LOGarithmic | PERCent | LDB", "Flags"={"OPC Wait"=FALSE, "Dont check status"=FALSE, "*WAI"=FALSE}, "Check Status Callback"=""}, {"Level"=2, "Descriptive Name"="Video Bandwidth", "Class Only"=FALSE, "Data Type"=1, "Access"=2, "Identifier"="RSZVL_ATTR_VIDEO_BANDWIDTH", "Range Table"="rszvl_rngVBW", "Command"="SENS:BAND:VID", "Read Callback"="", "Write Callback"="", "Range Callback"="", "Check Callback"="", "Rngtable Callback"="", "Coerce Callback"="", "User Callback"="", "Supported Models"="", "Instrument Options"="", "Repeated Capabilities"="", "Restricted Repeated Capabilities"="", "Help"="This attribute defines the instrument's video bandwidth.\n\nAvailable Repeated Capabilities:\nNone\n\nRemote-control command(s):\n[SENSe<1|2>:]BANDwidth|BWIDth:VIDeo", "Flags"={"OPC Wait"=FALSE, "Dont check status"=FALSE, "*WAI"=FALSE}, "Check Status Callback"=""}, {"Level"=2, "Descriptive Name"="Video Bandwidth Auto", "Class Only"=FALSE, "Data Type"=3, "Access"=2, "Identifier"="RSZVL_ATTR_VIDEO_BANDWIDTH_AUTO", "Range Table"="", "Command"="SENS:BAND:VID:AUTO", "Read Callback"="", "Write Callback"="", "Range Callback"="", "Check Callback"="", "Rngtable Callback"="", "Coerce Callback"="", "User Callback"="", "Supported Models"="", "Instrument Options"="", "Repeated Capabilities"="", "Restricted Repeated Capabilities"="", "Help"="This attribute either automatically couples the instrument's video bandwidth to the resolution bandwidth or cancels the coupling.\n\nAvailable Repeated Capabilities:\nNone\n\nRemote-control command(s):\n[SENSe<1|2>:]BANDwidth|BWIDth:VIDeo:AUTO ON | OFF", "Flags"={"OPC Wait"=FALSE, "Dont check status"=FALSE, "*WAI"=FALSE}, "Check Status Callback"=""}, {"Level"=2, "Descriptive Name"="Video Bandwidth Ratio", "Class Only"=FALSE, "Data Type"=1, "Access"=2, "Identifier"="RSZVL_ATTR_VIDEO_BANDWIDTH_RATIO", "Range Table"="rszvl_rngVbwRatio", "Command"="SENS:BAND:VID:RAT", "Read Callback"="", "Write Callback"="", "Range Callback"="", "Check Callback"="", "Rngtable Callback"="", "Coerce Callback"="", "User Callback"="", "Supported Models"="", "Instrument Options"="", "Repeated Capabilities"="", "Restricted Repeated Capabilities"="", "Help"="This attribute defines the ratio video bandwidth (Hz) / resolution bandwidth (Hz). The ratio to be entered is reciprocal to the ratio RBW/VBW used in manual control.\n\nAvailable Repeated Capabilities:\nNone\n\nRemote-control command(s):\n[SENSe<1|2>:]BANDwidth|BWIDth:VIDeo:RATio", "Flags"={"OPC Wait"=FALSE, "Dont check status"=FALSE, "*WAI"=FALSE}, "Check Status Callback"=""}, {"Level"=2, "Descriptive Name"="Low-Level Measurement", "Class Only"=TRUE, "Data Type"=0, "Access"=0, "Identifier"="", "Range Table"="", "Command"="", "Read Callback"="", "Write Callback"="", "Range Callback"="", "Check Callback"="", "Rngtable Callback"="", "Coerce Callback"="", "User Callback"="", "Supported Models"="", "Instrument Options"="", "Repeated Capabilities"="", "Restricted Repeated Capabilities"="", "Help"="This class contains attributes for initiate and abort measurement.\n\n(1) Abort:\nThis attribute aborts a current measurement and resets the trigger system.\n\n(2) Initiate:\nThis attribute initiates a new sweep.\nIn single sweep mode, synchronization to the end of the indicated number of measurements is achieved with the command *OPC. In continuous-sweep mode, synchronization to the sweep end is not possible since the overall measurement never ends.\n\n(3) Initiate Continuous:\nThis attribute determines whether the trigger system is continuously initiated (continuous) or performs single measurements (single).\nIn the spectrum analysis mode, this setting refers to the sweep sequence (switching between continuous/single sweep).\n\n(4) Send Software Trigger:\nThis attribute sends a software trigger to the instrument.\n\n(5) Continue Measurement:\nThis attribute continues 
